vi "Read Log After RSSI.vi"(6 "2.45 GHz Wake-Up Power":i8(ring)=6 items=["-29"=-29, "-4"=-4, "-2"=-2, "0"=0, "2"=2, "4"=4, "6"=6, "8"=8, "10"=10, "12"=12, "14"=14, "16"=16, "18"=18, "20"=20, "22"=22, "24"=24, "26"=26, "27"=27], 8 "error in":errorcluster, 9 "Attenuation dB (0)":dbl, 10 "400 MHz MICS Power Setting":u8=28 format="%.0x", 11 "VISA resource name":refnum<visa-resource-name>) -> (0 "error out":errorcluster, 1 "RSSI Values":u32[](array[numeric]), 2 "RSSI Values (String, HEX)":string[](array[string]), 3 "dup VISA Resource Name":refnum<visa-resource-name>)   [LabVIEW 2010]
uses:
  Typedef Command List.ctl
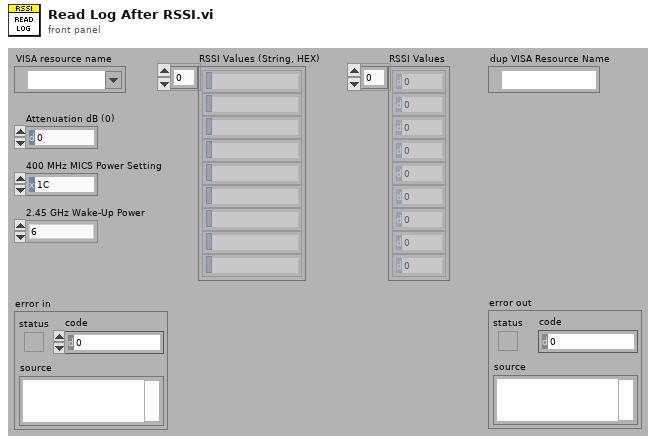
[diagram p1: front panel]
types:
  T1 = cluster{"Response Token":string, "Response Code":string, "bChecksum Valid":bool, "tChecksum Valid":bool, "CP_DATA OUT":u8[], "Data":string}
  T2 = typedef "Typedef Command List.ctl" = enum16{"Get xPG Status", "xPG Stimulation", "Select Program", "Increment Program Amplitude", "Decrement Program Amplitude", "Get PoP Constants", "Get PPC Constants", "Get Program Names", "Set Pulse Amplitude", "Increment Pulse Amplitude", "Decrement Pulse Amplitude", "Get Pulse Widths", "Set Pulse Widths", "Increment Pulse Width", "Decrement Pulse Width", "Get Program Frequency", "Set Program Frequency", "Increment Program Frequency", "Decrement Program Frequency", "Inject Event", "Charging Control", "Get xPG Identity", "Set xPG Identity", "Restore Program Defaults", "Get Program Definition", "Set Program Definition", "Get Program Constants", "Set Program Constants", "Get Configurable Device Parameters", "Set Configurable Device Parameters", "Get Pulse Constants", "Set Pulse Constants", "Get Lead Limits", "Set Lead Limits", "Get Channel Calibrations", "Set Channel Calibrations", "<reserved 2>", "<reserved 3>", "<reserved 4>", "<reserved 5>", "<reserved 6>", "<reserved 7>", "Get Stim Asic HV Calibrations", "Set Stim Asic HV Calibrations", "<reserved 8>", "<reserved 9>", "Get CP Data", "Set CP Data", "Clear Log", "Read Log", "Append Log", "Get Patient Program Runtime", "Set Patient Program Runtime", "Impedance Measurement", "Enter Storage Mode", "Echo Short", "Echo Long", "Get General Calibration", "Set General Calibration", "Get Trim List", "Set Trim List", "Get Counter", "Set Counter", "Get Test Stimulation", "Set Test Stimulation", "Get Titration Stimulation", "Set Titration Stimulation", "Get Ramp Time", "Set Ramp Time", "Get VBAT", "Set Software Description Block", "Get Software Description Block", "Write Memory", "Read Memory", "Reset xPG", "Erase Flash Block", "Write Vectors", "Read Vectors", "Diagnostic Data", "Set Background Impedance", "Get Background Impedence ", "Set Test Waveform", "Calibrate Channel", "Get Log Range", "Reserved 0x55", "Reserved 0x56", "MICS Options", "Pair PPC", "Pair POP", "Stop Bootloader", "Tune MICS", "MICS Diagnostics", "Undefined"}
  T3 = cluster{"Command":T2, "Function":enum16{"Open Session", "Close Session", "Downlink Only", "Uplink Only", "Transceive (DN -> UP)"}, "MICS_ID":u32, "EXID":u32, "Use Local":bool, "Transceive Delay mS":dbl, "CP_DATA IN":u8[], "Parameters":string}
  T4 = enum16{"Get Device Type", "Get Device Name", "Get Device Version", "Get Device Error"}
  T5 = cluster{"ERROR_OCCURRED":bool, "LINK_STAT_CHANGED":bool, "LINK_QUAL_CHANGED":bool, "400MHZ_TX_ACTIVE":bool, "400MHZ_RX_ACTIVE":bool, "245GHZ_TX_ACTIVE":bool, "DATA_STAT_CHANGED":bool, "SLEEPING":bool, "IDLE":bool, "SEARCHING_FOR_IMPLANT":bool, "STARTING_SESSION":bool, "LISTENING_FOR_EMERG":bool, "IN_SESSION":bool}
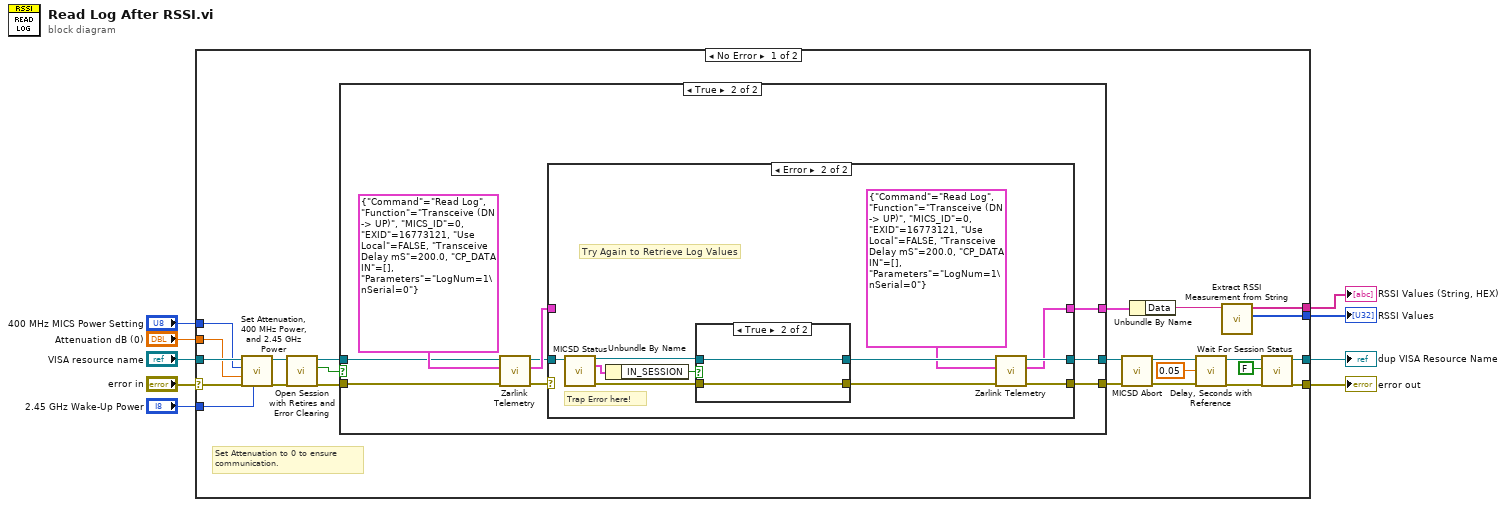
[diagram p0: block diagram]
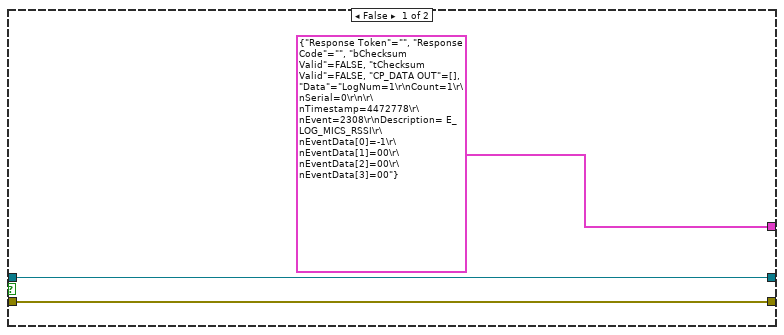
[diagram p2: hidden frame]
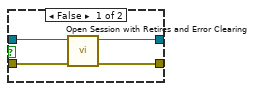
[diagram p4: hidden frame]
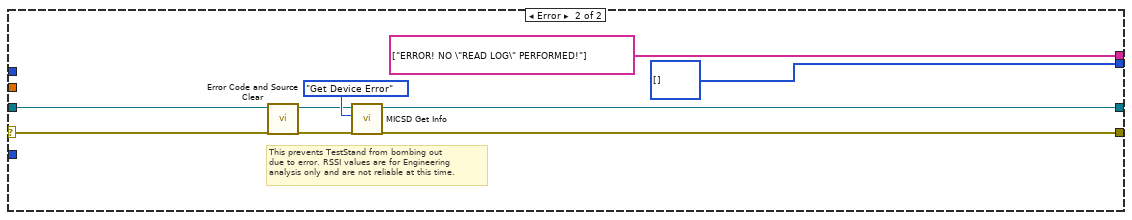
[diagram p5: hidden frame]
diagram:
  n1 = case shown="No Error" "error in" {
    selector: "error in" -> [w15 w67]
    tunnel: [w32 u32[] [] ("RSSI Values")] -> w9
    tunnel: [w31 string[] ["ERROR! NO \"READ LOG\" PERFORMED!"] ("RSSI Values (String, HEX)")] -> w8
    tunnel: "VISA resource name" -> [w29 w65]
    tunnel: "400 MHz MICS Power Setting" -> [w28 _]
    tunnel: "Attenuation dB (0)" -> [w27 _]
    tunnel: [w23 w64] -> w4
    tunnel: [w22 w66] -> w3
    tunnel: "2.45 GHz Wake-Up Power" -> [w21 _]
    frame No Error {
      # "Set Attenuation to 0 to ensure\ncommunication."
      n2 = call "Set Attenuation, 400 MHz Power, and 2.45 GHz Power.vi"("2.45 GHz Wake-Up Power (6)"=w21, "error in"=w15, "Attenuation dB (0)"=w27, "400 MHz MICS Power Setting (0x16)"=w28, "VISA Resource Name"=w29) -> ("error out"=w18:errorcluster, "dup VISA Resource Name"=w20:refnum<visa-resource-name>)  [unwired: 5 in]
      n3 = call "Open Session with Retires and Error Clearing.vi"("error in"=w18, "VISA Resource Name"=w20) -> ("error out"=w17:errorcluster, "IN_SESSION"=w16:bool, "dup VISA Resource Name"=w19:refnum<visa-resource-name>)  [unwired: 6 in, 1 out]
      n4 = case shown="True" w16 {
        tunnel: [T1 {"Response Token"="", "Response Code"="", "bChecksum Valid"=FALSE, "tChecksum Valid"=FALSE, "CP_DATA OUT"=[], "Data"="LogNum=1\r\nCount=1\r\nSerial=0\r\n\r\nTimestamp=4472778\r\nEvent=2308\r\nDescription= E_LOG_MICS_RSSI\r\nEventData[0]=-1\r\nEventData[1]=00\r\nEventData[2]=00\r\nEventData[3]=00"} ("Output") w43] -> w33
        tunnel: [w34 w40] -> w26
        tunnel: [w35 w39] -> w25
        tunnel: w19 -> [w34 w38]
        tunnel: w17 -> [w35 w37]
        frame False {
        }
        frame True {
          n5 = call "Zarlink Telemetry.vi"("error in (no error)"=w37, "Input"=T3 {"Command"=enum."Read Log", "Function"=enum."Transceive (DN -> UP)", "MICS_ID"=0, "EXID"=16773121, "Use Local"=FALSE, "Transceive Delay mS"=200.0, "CP_DATA IN"=[], "Parameters"="LogNum=1\nSerial=0"}, "MICS Dongle Address"=w38) -> ("error out"=w44:errorcluster, "Output"=w42:T1)  [unwired: 6 in, 1 out]
          n6 = case shown="Error" w44 {
            selector: w44 -> [w46 _]
            tunnel: w42 -> [w47 _]
            tunnel: [w47 w50] -> w43
            tunnel: [w45 w51] -> w40
            tunnel: [w46 w53] -> w39
            tunnel: w38 -> [w45 w48]
            frame No Error {
            }
            frame Error {
              # "Try Again to Retrieve Log Values"
              # "Trap Error here!"
              n7 = call "MICSD Status.vi"() -> ()  [unwired: 9 in, 7 out]
              n8 = call "MICSD Status.vi"("VISA Resource Name"=w48) -> ("dup VISA Resource Name"=w54:refnum<visa-resource-name>, "Status Flags"=w57:T5, "error out"=w55:errorcluster)  [unwired: 8 in, 4 out]
              n9 = Unbundle By Name(w57) -> ("IN_SESSION"=w56:bool)
              n10 = case shown="True" w56 {
                tunnel: w54 -> [w61 w63]
                tunnel: [w60 w63] -> w51
                tunnel: w55 -> [w59 w62]
                tunnel: [w58 w62] -> w52
                frame False {
                  n11 = call "Open Session with Retires and Error Clearing.vi"("error in"=w59, "VISA Resource Name"=w61) -> ("error out"=w58:errorcluster, "dup VISA Resource Name"=w60:refnum<visa-resource-name>)  [unwired: 6 in, 2 out]
                }
                frame True {
                }
              }
              n12 = call "Zarlink Telemetry.vi"("error in (no error)"=w52, "Input"=T3 {"Command"=enum."Read Log", "Function"=enum."Transceive (DN -> UP)", "MICS_ID"=0, "EXID"=16773121, "Use Local"=FALSE, "Transceive Delay mS"=200.0, "CP_DATA IN"=[], "Parameters"="LogNum=1\nSerial=0"}, "MICS Dongle Address"=w51) -> ("error out"=w53:errorcluster, "Output"=w50:T1)  [unwired: 6 in, 1 out]
            }
          }
        }
      }
      n13 = call "MICSD Abort.vi"("error in (no error)"=w25, "VISA Resource Name"=w26) -> ("error out"=w12:errorcluster, "dup VISA Resource Name"=w14:refnum<visa-resource-name>)  [unwired: 8 in]
      n14 = Unbundle By Name(w33) -> ("Data"=w30:string)
      n15 = call "Delay, Seconds with Reference.vi"("error in"=w12, "delay"=dbl[unit] 0.05, "VISA resource"=w14) -> ("error out"=w11:errorcluster, "VISA resource dup"=w13:refnum<visa-resource-name>)  [unwired: 3 in, 1 out]
      n16 = call "Extract RSSI Measurement from String.vi"("Normal Event Log String"=w30) -> ("RSSI Values"=w32:u32[], "RSSI Values (String, HEX)"=w31:string[])  [unwired: 9 in]
      n17 = call "Wait For Session Status.vi"("error in (no error)"=w11, "IN_SESSION State (T)"=FALSE, "VISA Resource Name"=w13) -> ("error out"=w22:errorcluster, "dup VISA Resource Name"=w23:refnum<visa-resource-name>)  [unwired: 5 in, 2 out]
    }
    frame Error {
      # "This prevents TestStand from bombing out\ndue to error. RSSI values are for Engineering\nanalysis only and are not reliable at this time."
      n18 = call "Error Code and Source Clear.vi"("error in"=w67) -> ("error out"=w68:errorcluster)  [unwired: 8 in]
      n19 = call "MICSD Get Info.vi"("error in (no error)"=w68, "Command"=T4."Get Device Error", "VISA Resource Name"=w65) -> ("error out"=w66:errorcluster, "dup VISA Resource Name"=w64:refnum<visa-resource-name>)  [unwired: 6 in, 1 out]
    }
  }
  "error out" <- w3
  "dup VISA Resource Name" <- w4
  "RSSI Values" <- w9
  "RSSI Values (String, HEX)" <- w8
